vi "TCP Send with CRLF.vi"(0 "CART TCP Connection":refnum<k5>, 7 "data in":string, 11 "error IO":errorcluster) -> (4 "CART TCP Connection Out":refnum<k5>, 15 "error out":errorcluster)   [LabVIEW 2012]
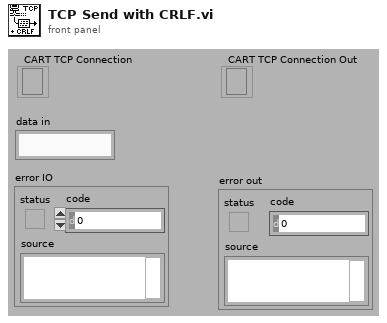
[diagram p1: front panel]
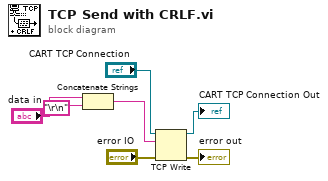
[diagram p0: block diagram]
diagram:
  n1 = Concatenate Strings("data in", "\r\n") -> (w6:string)
  n2 = TCP Write(connection ID="CART TCP Connection", data in=w6, error in (no error)="error IO") -> (connection ID out=→"CART TCP Connection Out":refnum<k5>, error out=→"error out":errorcluster)  [unwired: 1 in, 1 out]
